vi "NotifyRegistered.vi"(2 "data string":string, 3 "ROS":T1={"topic port"=0, "Node"="", "topic"="", "type"="", "node port"=0, "error "={"status"=FALSE, "code"=0, "source"=""}, "Direction"=enum."Node", "APIs"=[], "Update (ms)"=1, "write queue"=1}) -> ()   [LabVIEW 2010]
uses:
  SubVIs/_ROSDirection.ctl
  SubVIs/_ROSControl.ctl
panel:
  out "vi name":string
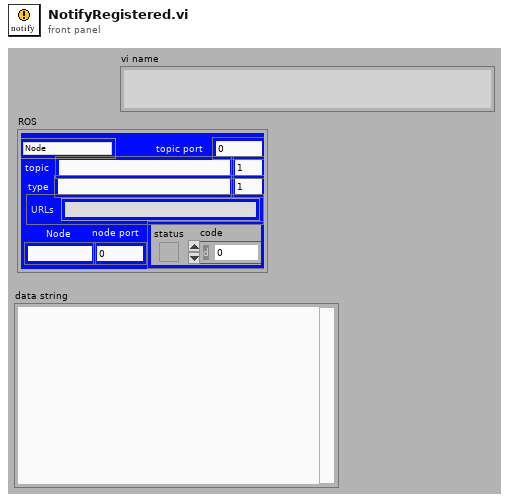
[diagram p1: front panel]
types:
  T1 = typedef "_ROSControl.ctl" = cluster{"topic port":u16, "Node":string, "topic":string, "type":string, "node port":u32, "error ":errorcluster, "Direction":T2, "APIs":string[], "Update (ms)":u16, "write queue":u16}
  T2 = typedef "_ROSDirection.ctl" = enum16{"Node", "Publisher", "Subscriber", "Service Client"}
  T3 = typedef "ServoInfo.ctl" = cluster{"vi name":string, "VI Refnum":refnum<vi>, "queue":refnum<queue>, "ROS":T1, "notifier":refnum<notifier>}
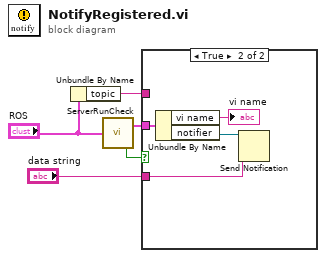
[diagram p0: block diagram]
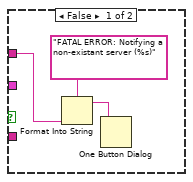
[diagram p2: hidden frame]
diagram:
  n1 = Unbundle By Name("ROS") -> ("topic"=w1:string)
  n2 = call "ServerRunCheck.vi"("ROS in"="ROS") -> ("Running?"=w3:bool, "ServerFound"=w4:T3)
  n3 = case shown="True" w3 {
    tunnel: "data string" -> [_ w12]
    tunnel: w4 -> [_ w11]
    tunnel: w1 -> [w6 _]
    frame False {
      n4 = Format Into String(format string="FATAL ERROR: Notifying a non-existant server (%s)" ("message"), w6) -> (resulting string=w8:string)  [unwired: 2 in, 1 out]
      n5 = One Button Dialog(message=w8) -> ()  [unwired: 1 in, 1 out]
    }
    frame True {
      n6 = Unbundle By Name(w11) -> ("vi name"=→"vi name":string, "notifier"=w10:refnum<notifier>)
      n7 = Send Notification(notification=w12, notifier=w10) -> ()  [unwired: 1 in, 2 out]
    }
  }
